vi "Read Colors.vi"(9 "Page in":refnum<class "Page.lvclass">) -> (3 "Page out":refnum<class "Page.lvclass">, 4 "Colors":T1)   [LabVIEW 2014, in "Raspberry Pi Compatible Compiler for LabVIEW.lvlib" / "Page.lvclass"]
uses:
  Page.lvclass
  <vilib>/Utility/miscctls.llb/LVForegroundBackgroundColorsTypeDef.ctl
  Page.lvclass/Page.ctl
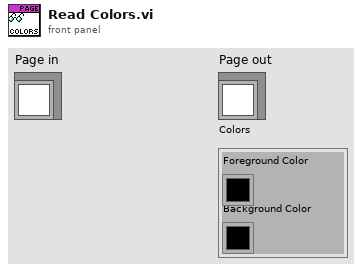
[diagram p1: front panel]
types:
  T1 = typedef "LVForegroundBackgroundColorsTypeDef.ctl" = cluster{"Foreground Color":u32, "Background Color":u32}
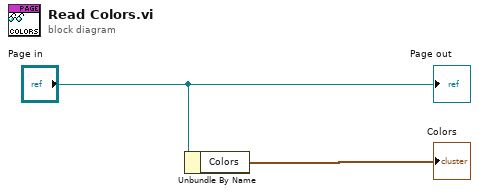
[diagram p0: block diagram]
diagram:
  n1 = Unbundle By Name("Page in") -> ("Colors"=→"Colors":T1)
  "Page out" <- "Page in"
